vi "getKeyFormatAndRowChkRes.vi"(5 "keyVal":string, 6 "keyName":string, 7 "section":string, 8 "error in":errorcluster, 9 "Row number":u32, 10 "table":string[][](array[string]), 11 "Tree Refnum in":refnum<vi>) -> (0 "error out":errorcluster, 1 "chkRes":string="√", 2 "keyFormat":string, 3 "Tree Refnum out":refnum<vi>)   [LabVIEW 2010]
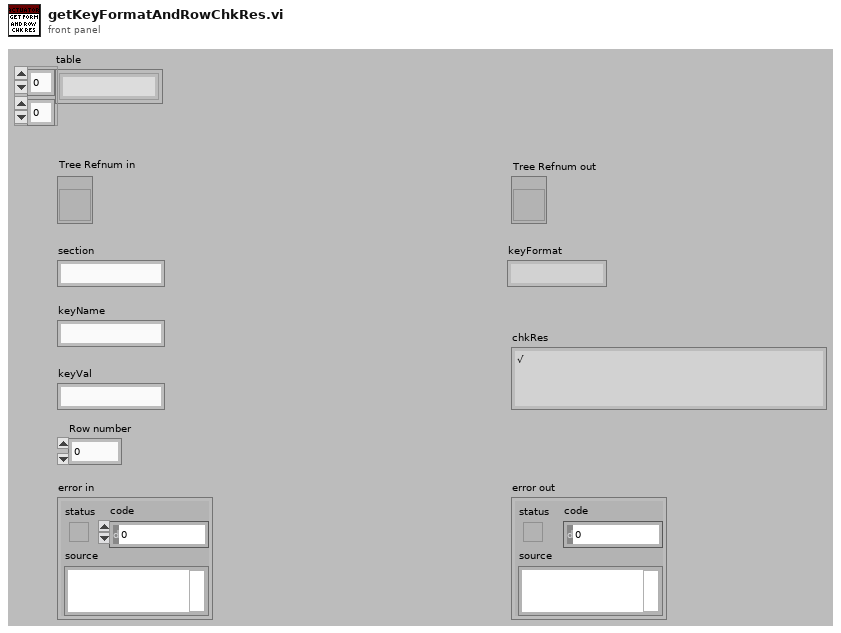
[diagram p1: front panel]
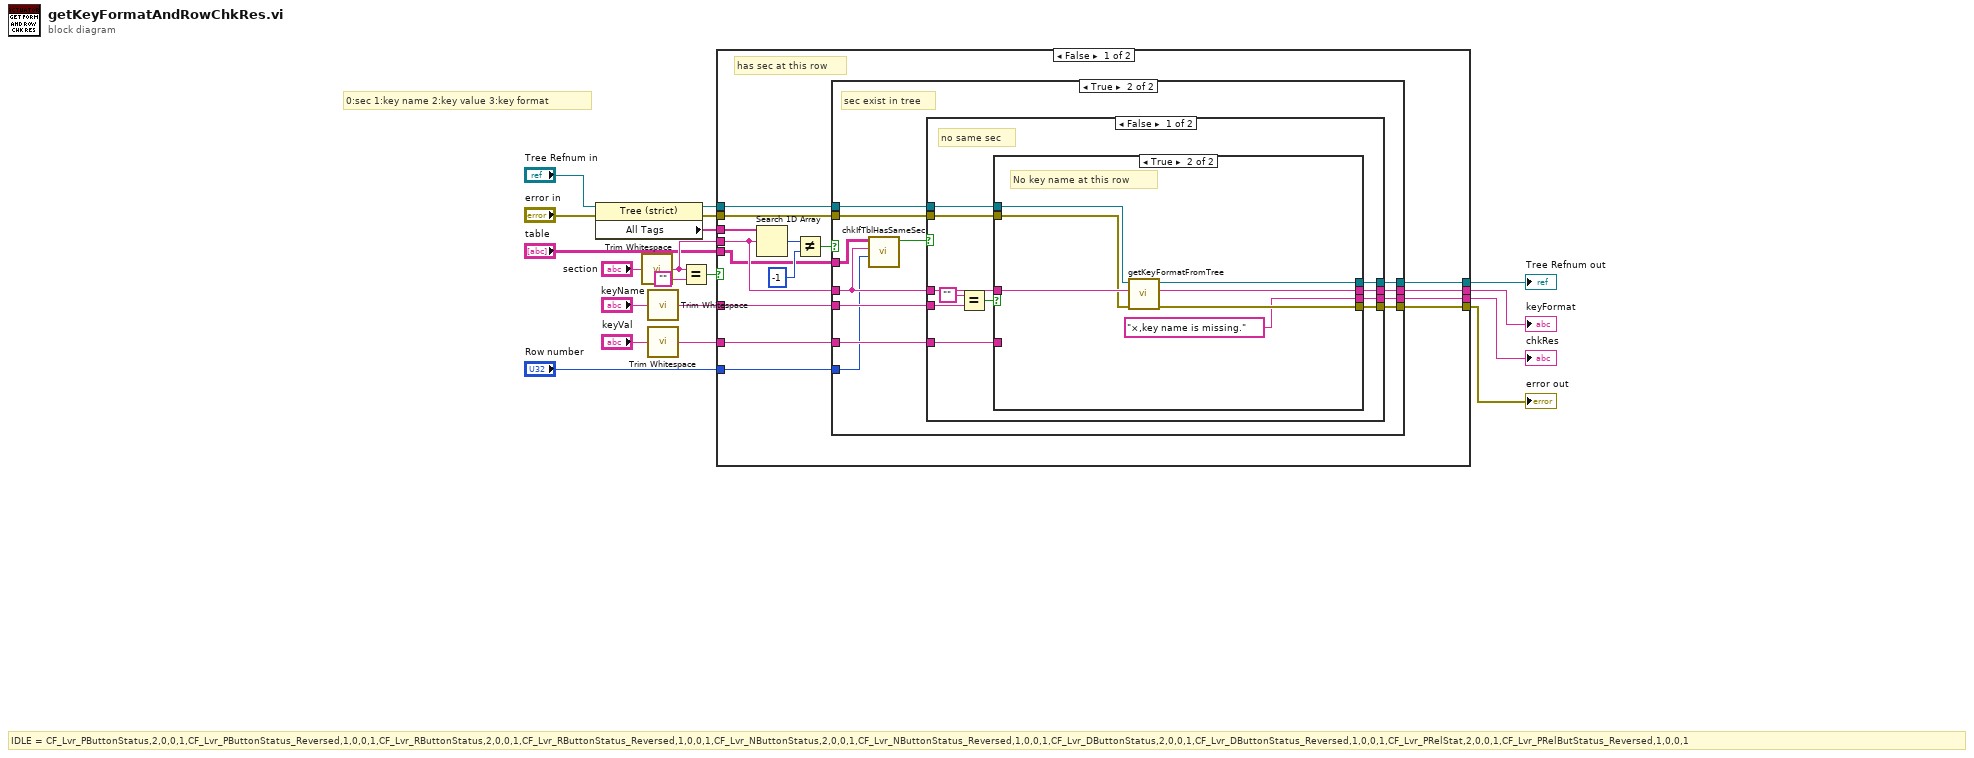
[diagram p0: block diagram]
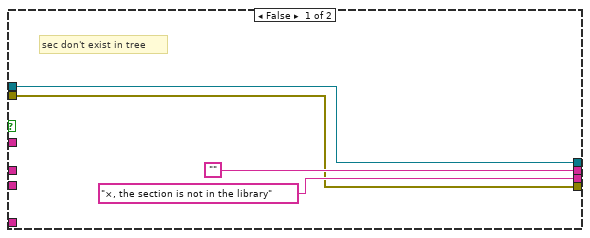
[diagram p2: hidden frame]
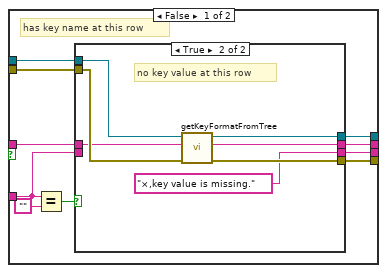
[diagram p3: hidden frame]
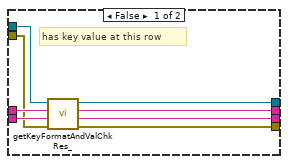
[diagram p4: hidden frame]
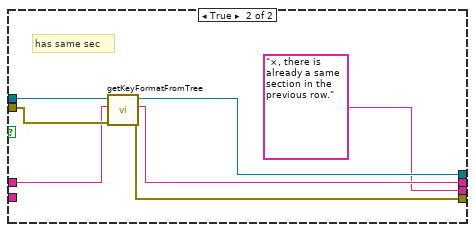
[diagram p5: hidden frame]
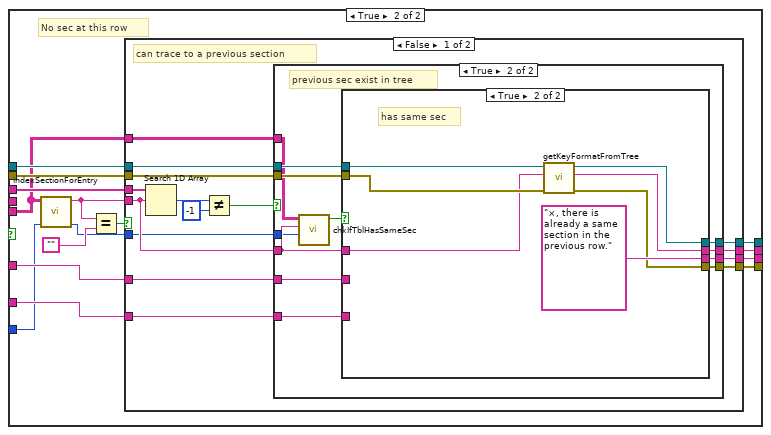
[diagram p6: hidden frame]
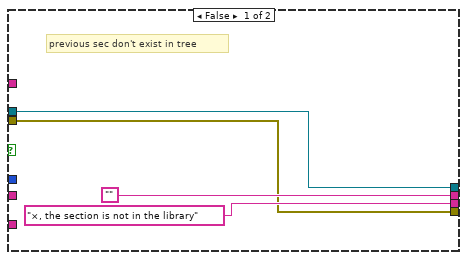
[diagram p7: hidden frame]
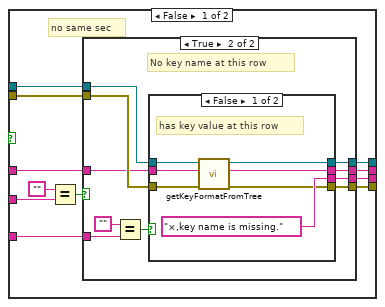
[diagram p8: hidden frame]
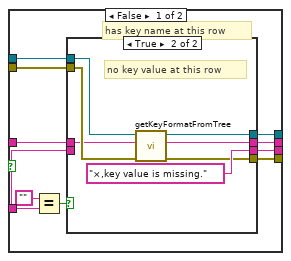
[diagram p9: hidden frame]
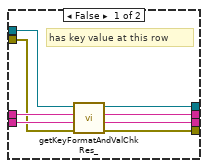
[diagram p10: hidden frame]
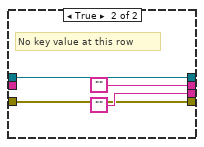
[diagram p11: hidden frame]
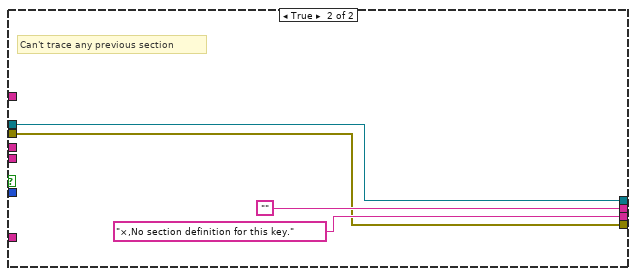
[diagram p12: hidden frame]
diagram:
  # "IDLE = CF_Lvr_PButtonStatus,2,0,0,1,CF_Lvr_PButtonStatus_Reversed,1,0,0,1,CF_Lvr_RButtonStatus,2,0,0,1,CF_Lvr_RButtonStatus_Reversed,1,0,0,1,CF_Lvr_NButtonStatus,2,0,0,1,CF_Lvr_NButtonStatus_Reversed,1,0,0,1,CF_Lvr_DButtonStatus,2,0,0,1,CF_Lvr_DButtonStatus_Reversed,1,0,0,1,CF_Lvr_PRelStat,2,0,0,1,CF_Lvr_PRelButStatus_Reversed,1,0,0,1"
  # "0:sec 1:key name 2:key value 3:key format"
  n1 = property on="Property Node" class="Tree (strict)"(reference="Tree Refnum in", error in="error in") -> (reference out=w13:refnum<vi>, error out=w12:errorcluster, "All Tags"=w16:string[])
  n2 = call <vilib>:"Trim Whitespace.vi"("string"="section") -> ("trimmed string"=w11:string)  [unwired: 1 in]
  n3 = call <vilib>:"Trim Whitespace.vi"("string"="keyName") -> ("trimmed string"=w15:string)  [unwired: 1 in]
  n4 = call <vilib>:"Trim Whitespace.vi"("string"="keyVal") -> ("trimmed string"=w14:string)  [unwired: 1 in]
  n5 = Equal?(x=w11, y="") -> (x = y?=w18:bool)
  n6 = case shown="False" w18 {
    tunnel: w16 -> [w34 w113]
    tunnel: w15 -> [w30 w112]
    tunnel: w14 -> [w29 w111]
    tunnel: w13 -> [w28 w110]
    tunnel: w12 -> [w26 w109]
    tunnel: w11 -> [w27 _]
    tunnel: [w23 w108] -> w10
    tunnel: [w24 w107] -> w2
    tunnel: [w25 w106] -> w9
    tunnel: [w22 w105] -> w1
    tunnel: "table" -> [w20 w102]
    tunnel: "Row number" -> [w21 w103]
    frame False {
      # "has sec at this row"
      n7 = Search 1D Array(1D array=w34, element=w27) -> (index of element=w33:i32)  [unwired: 1 in]
      n8 = Not Equal?(x=w33, y=-1) -> (x != y?=w31:bool)
      n9 = case shown="True" w31 {
        tunnel: w30 -> [_ w50]
        tunnel: w29 -> [_ w49]
        tunnel: w28 -> [w35 w48]
        tunnel: w27 -> [_ w43]
        tunnel: w26 -> [w36 w47]
        tunnel: ["×, the section is not in the library" w39] -> w25
        tunnel: ["" w46] -> w24
        tunnel: [w35 w45] -> w23
        tunnel: [w36 w44] -> w22
        tunnel: w21 -> [_ w42]
        tunnel: w20 -> [_ w41]
        frame False {
          # "sec don't exist in tree"
        }
        frame True {
          # "sec exist in tree"
          n10 = call "chkIfTblHasSameSec.vi"("rowNumAtWhichSecExist"=w42, "Section"=w43, "tbl"=w41) -> ("foundSameSec?"=w40:bool)  [unwired: 8 in]
          n11 = case shown="False" w40 {
            tunnel: w50 -> [w61 _]
            tunnel: w49 -> [w58 _]
            tunnel: w48 -> [w57 w100]
            tunnel: w47 -> [w56 w99]
            tunnel: [w54 w97] -> w46
            tunnel: [w53 w96] -> w45
            tunnel: [w52 w95] -> w44
            tunnel: w43 -> [w51 w98]
            tunnel: [w55 "×, there is already a same section in the previous row."] -> w39
            frame False {
              # "no same sec"
              n12 = Equal?(x="", y=w61) -> (x = y?=w59:bool)
              n13 = case shown="True" w59 {
                tunnel: w58 -> [w67 _]
                tunnel: w57 -> [w70 w92]
                tunnel: w51 -> [w69 w91]
                tunnel: w56 -> [w66 w90]
                tunnel: [w65 "×,key name is missing."] -> w55
                tunnel: [w64 w93] -> w54
                tunnel: [w63 w87] -> w53
                tunnel: [w62 w89] -> w52
                frame False {
                  # "has key name at this row"
                  n14 = Equal?(x=w67, y="") -> (x = y?=w71:bool)
                  n15 = case shown="True" w71 {
                    tunnel: w70 -> [w79 w83]
                    tunnel: w69 -> [w78 w82]
                    tunnel: w67 -> [w77 _]
                    tunnel: w66 -> [w76 w84]
                    tunnel: [w75 "×,key value is missing."] -> w65
                    tunnel: [w74 w86] -> w64
                    tunnel: [w73 w81] -> w63
                    tunnel: [w72 w85] -> w62
                    frame False {
                      # "has key value at this row"
                      n16 = call "getKeyFormatAndValChkRes_.vi"("error in"=w76, "keyVal"=w77, "sec"=w78, "Tree Refnum in"=w79) -> ("error out"=w72:errorcluster, "chkRes"=w75:string, "keyFormat"=w74:string, "Tree Refnum out"=w73:refnum<vi>)  [unwired: 4 in]
                    }
                    frame True {
                      # "no key value at this row"
                      n17 = call "getKeyFormatFromTree.vi"("error in"=w84, "sec"=w82, "Tree Refnum in"=w83) -> ("error out"=w85:errorcluster, "keyFormat"=w86:string, "Tree Refnum out"=w81:refnum<vi>)  [unwired: 6 in]
                    }
                  }
                }
                frame True {
                  # "No key name at this row"
                  n18 = call "getKeyFormatFromTree.vi"("error in"=w90, "sec"=w91, "Tree Refnum in"=w92) -> ("error out"=w89:errorcluster, "keyFormat"=w93:string, "Tree Refnum out"=w87:refnum<vi>)  [unwired: 6 in]
                }
              }
            }
            frame True {
              # "has same sec"
              n19 = call "getKeyFormatFromTree.vi"("error in"=w99, "sec"=w98, "Tree Refnum in"=w100) -> ("error out"=w95:errorcluster, "keyFormat"=w97:string, "Tree Refnum out"=w96:refnum<vi>)  [unwired: 6 in]
            }
          }
        }
      }
    }
    frame True {
      # "No sec at this row"
      n20 = call "indexSectionForEntry.vi"("rowNum"=w103, "tbl"=w102) -> ("rowNumAtWhichSecExist"=w101:i32, "indexSection"=w104:string)  [unwired: 8 in]
      n21 = Equal?(x=w104, y="") -> (x = y?=w114:bool)
      n22 = case shown="False" w114 {
        tunnel: w113 -> [w128 _]
        tunnel: w104 -> [w123 _]
        tunnel: w112 -> [w126 _]
        tunnel: w111 -> [w125 _]
        tunnel: w110 -> [w124 w211]
        tunnel: w109 -> [w122 w212]
        tunnel: [w121 w211] -> w108
        tunnel: [w120 ""] -> w107
        tunnel: [w119 "×,No section definition for this key."] -> w106
        tunnel: [w118 w212] -> w105
        tunnel: w102 -> [w117 _]
        tunnel: w101 -> [w116 _]
        frame False {
          # "can trace to a previous section"
          n23 = Search 1D Array(1D array=w128, element=w123) -> (index of element=w129:i32)  [unwired: 1 in]
          n24 = Not Equal?(x=w129, y=-1) -> (x != y?=w127:bool)
          n25 = case shown="True" w127 {
            tunnel: w126 -> [_ w146]
            tunnel: w125 -> [_ w145]
            tunnel: w124 -> [w134 w144]
            tunnel: w123 -> [_ w138]
            tunnel: w122 -> [w131 w143]
            tunnel: [w134 w142] -> w121
            tunnel: ["" w141] -> w120
            tunnel: ["×, the section is not in the library" w140] -> w119
            tunnel: [w131 w139] -> w118
            tunnel: w117 -> [_ w137]
            tunnel: w116 -> [_ w135]
            frame False {
              # "previous sec don't exist in tree"
            }
            frame True {
              # "previous sec exist in tree"
              n26 = call "chkIfTblHasSameSec.vi"("rowNumAtWhichSecExist"=w135, "Section"=w138, "tbl"=w137) -> ("foundSameSec?"=w136:bool)  [unwired: 8 in]
              n27 = case shown="True" w136 {
                tunnel: w146 -> [w157 _]
                tunnel: w145 -> [w154 _]
                tunnel: w144 -> [w153 w207]
                tunnel: w143 -> [w152 w206]
                tunnel: [w151 w208] -> w142
                tunnel: [w150 w209] -> w141
                tunnel: [w149 "×, there is already a same section in the previous row."] -> w140
                tunnel: [w148 w205] -> w139
                tunnel: w138 -> [w147 w204]
                frame False {
                  # "no same sec"
                  n28 = Equal?(x="", y=w157) -> (x = y?=w155:bool)
                  n29 = case shown="True" w155 {
                    tunnel: w154 -> [w163 w192]
                    tunnel: w153 -> [w165 w184]
                    tunnel: w147 -> [w164 w183]
                    tunnel: w152 -> [w162 w187]
                    tunnel: [w161 w185] -> w151
                    tunnel: [w160 w189] -> w150
                    tunnel: [w159 w188] -> w149
                    tunnel: [w158 w186] -> w148
                    frame False {
                      # "has key name at this row"
                      n30 = Equal?(x="", y=w163) -> (x = y?=w166:bool)
                      n31 = case shown="True" w166 {
                        tunnel: w165 -> [w175 w179]
                        tunnel: w164 -> [w174 w180]
                        tunnel: w163 -> [w173 _]
                        tunnel: w162 -> [w172 w181]
                        tunnel: [w171 w178] -> w161
                        tunnel: [w170 w177] -> w160
                        tunnel: [w169 "×,key value is missing."] -> w159
                        tunnel: [w168 w176] -> w158
                        frame False {
                          # "has key value at this row"
                          n32 = call "getKeyFormatAndValChkRes_.vi"("error in"=w172, "keyVal"=w173, "sec"=w174, "Tree Refnum in"=w175) -> ("error out"=w168:errorcluster, "chkRes"=w169:string, "keyFormat"=w170:string, "Tree Refnum out"=w171:refnum<vi>)  [unwired: 4 in]
                        }
                        frame True {
                          # "no key value at this row"
                          n33 = call "getKeyFormatFromTree.vi"("error in"=w181, "sec"=w180, "Tree Refnum in"=w179) -> ("error out"=w176:errorcluster, "keyFormat"=w177:string, "Tree Refnum out"=w178:refnum<vi>)  [unwired: 6 in]
                        }
                      }
                    }
                    frame True {
                      # "No key name at this row"
                      n34 = Equal?(x="", y=w192) -> (x = y?=w190:bool)
                      n35 = case shown="False" w190 {
                        tunnel: [w196 ""] -> w189
                        tunnel: ["×,key name is missing." ""] -> w188
                        tunnel: w187 -> [w198 w201]
                        tunnel: [w197 w201] -> w186
                        tunnel: [w195 w200] -> w185
                        tunnel: w184 -> [w194 w200]
                        tunnel: w183 -> [w193 _]
                        frame False {
                          # "has key value at this row"
                          n36 = call "getKeyFormatFromTree.vi"("error in"=w198, "sec"=w193, "Tree Refnum in"=w194) -> ("error out"=w197:errorcluster, "keyFormat"=w196:string, "Tree Refnum out"=w195:refnum<vi>)  [unwired: 6 in]
                        }
                        frame True {
                          # "No key value at this row"
                        }
                      }
                    }
                  }
                }
                frame True {
                  # "has same sec"
                  n37 = call "getKeyFormatFromTree.vi"("error in"=w206, "sec"=w204, "Tree Refnum in"=w207) -> ("error out"=w205:errorcluster, "keyFormat"=w209:string, "Tree Refnum out"=w208:refnum<vi>)  [unwired: 6 in]
                }
              }
            }
          }
        }
        frame True {
          # "Can't trace any previous section"
        }
      }
    }
  }
  "error out" <- w1
  "Tree Refnum out" <- w10
  "chkRes" <- w9
  "keyFormat" <- w2
